vi "write_ini.vi"(8 "error in (no error)":errorcluster caption="错误输入（无错误）", 9 "section name":string, 10 "file ref in":T1, 11 "LimitSwitch 输入":refnum<class "LimitSwitch.lvclass">) -> (0 "error out":errorcluster caption="错误输出", 2 "file ref out":T1, 3 "LimitSwitch 输出":refnum<class "LimitSwitch.lvclass">)   [LabVIEW 2016, in "MotionControl.lvlib" / "LimitSwitch.lvclass"]
uses:
  <userlib>/MotionControl/LimitSwitch/LimitSwitch.lvclass
  <vilib>/Utility/config.llb/Config Data RefNum.ctl
  <userlib>/MotionControl/LimitSwitch/LimitSwitch.lvclass/LimitSwitch.ctl
  <vilib>/Utility/config.llb/Write Key (U32).vi
  <vilib>/Utility/config.llb/Write Key (I32).vi
  <vilib>/Utility/error.llb/Error Cluster From Error Code.vi
  <vilib>/ErrorRing/Error Ring.xnode
  <vilib>/Utility/config.llb/NI_LVConfig.lvlib
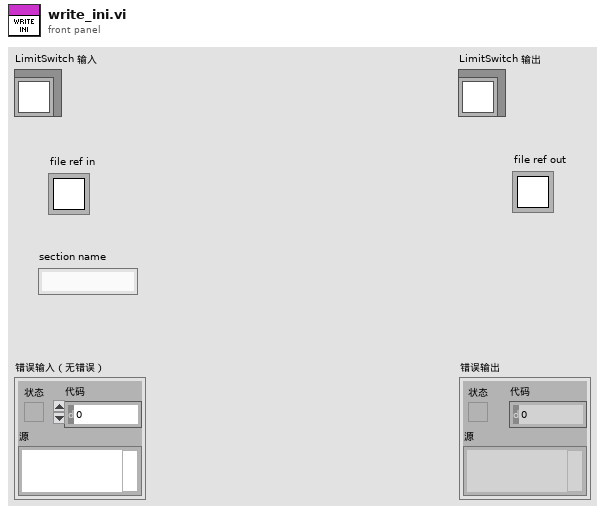
[diagram p1: front panel]
types:
  T1 = typedef "NI_LVConfig.lvlib/Config Data RefNum.ctl" = refnum<k1>
  T2 = typedef "MotionControl.lvlib/LimitSwitch.lvclass/LM_ID.ctl" = i32
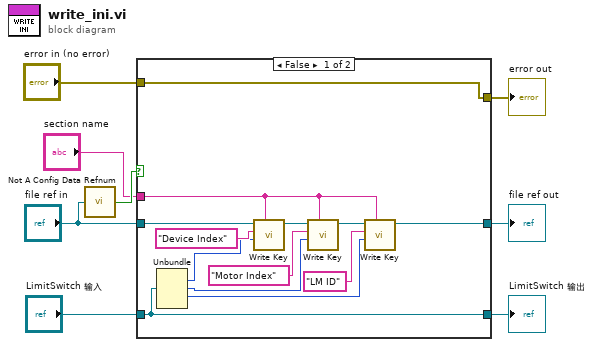
[diagram p0: block diagram]
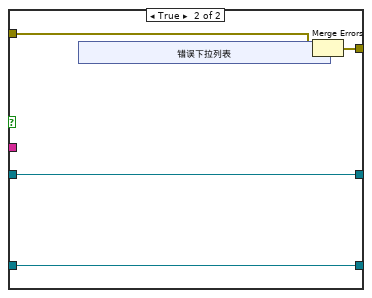
[diagram p2: hidden frame]
diagram:
  n1 = call <vilib>:"Not A Config Data Refnum.vi"("refnum"="file ref in") -> ("not a config data refnum"=w5:bool)
  n2 = case shown="False" w5 {
    tunnel: [w21 w23] -> w8
    tunnel: [w18 w26] -> w6
    tunnel: "LimitSwitch 输入" -> [w18 w26]
    tunnel: "error in (no error)" -> [w21 w24]
    tunnel: "file ref in" -> [w20 w22]
    tunnel: "section name" -> [w14 _]
    tunnel: [w9 w22] -> w1
    frame False {
      n3 = Unbundle(w18) -> (w17:u32, w12:u32, w10:T2)  [unwired: 2 out]
      n4 = call-poly <vilib>:"Write Key.vi"("section"=w14, "value"=w17, "key"="Device Index", "refnum"=w20) -> ("refnum out"=w16:T1)  [unwired: 5 in, 2 out]
      n5 = call-poly <vilib>:"Write Key.vi"("section"=w14, "value"=w12, "key"="Motor Index", "refnum"=w16) -> ("refnum out"=w15:T1)  [unwired: 5 in, 2 out]
      n6 = call-poly <vilib>:"Write Key.vi"("section"=w14, "value"=w10, "key"="LM ID", "refnum"=w15) -> ("refnum out"=w9:T1)  [unwired: 5 in, 2 out]
    }
    frame True {
      n7 = xnode "错误下拉列表"() -> ("error out"=w25:errorcluster)
      n8 = Merge Errors(w24, w25) -> (w23:errorcluster)
    }
  }
  "error out" <- w8
  "LimitSwitch 输出" <- w6
  "file ref out" <- w1
